vi "Configure Edge Trigger Coupling.vi"(0 "VISA resource name":refnum<visa-resource-name>, 5 "Edge Trigger Coupling (0: AC)":i32(ring) items=["AC", "DC", "Low Frequency Noise Reject", "High Frequency Noise Reject"], 11 "error in (no error)":errorcluster) -> (4 "VISA resource name out":refnum<visa-resource-name>, 15 "error out":errorcluster)   [LabVIEW 2013, in "Agilent 90000 Series.lvlib"]
doc: "Configures the coupling of edge trigger. Call <B>Configure Trigger (Edge) VI</B> to set the trigger mode to edge.\n\n<B>Notes:</B>\nThis VI is only available for 9k series."
uses:
  Agilent 90000 Series.lvlib
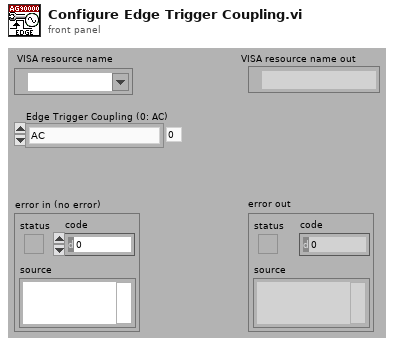
[diagram p1: front panel]
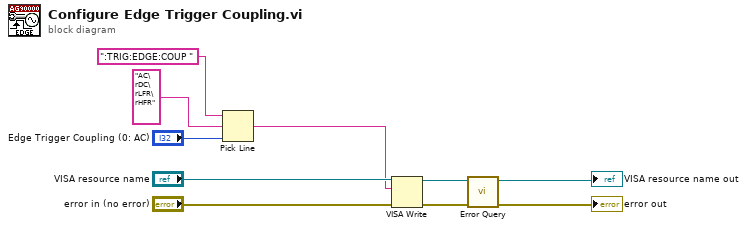
[diagram p0: block diagram]
diagram:
  n1 = Pick Line(string ("")=":TRIG:EDGE:COUP ", multi-line string="AC\rDC\rLFR\rHFR", line index="Edge Trigger Coupling (0: AC)") -> (output string=w1:string)
  n2 = VISA Write(VISA resource name="VISA resource name", write buffer=w1, error in (no error)="error in (no error)") -> (VISA resource name out=w6:refnum<visa-resource-name>, error out=w5:errorcluster)  [unwired: 1 out]
  n3 = call "Error Query.vi"("error in (no error)"=w5, "VISA resource name"=w6) -> ("error out"=→"error out":errorcluster, "VISA resource name out"=→"VISA resource name out":refnum<visa-resource-name>)  [unwired: 8 out]
